vi "Destroy.vi"(8 "error in (no error)":errorcluster, 11 "Server in":refnum<class "Server.lvclass">) -> (0 "error out":errorcluster, 3 "Server out":refnum<class "Server.lvclass">)   [LabVIEW 2013, in "MQTT Server.lvlib" / "Server.lvclass"]
uses:
  Server.lvclass
  MQTT_Base/MQTT_Base.lvclass
  Server.lvclass/Server.ctl
  StoredSessions/StoredSessions.lvclass
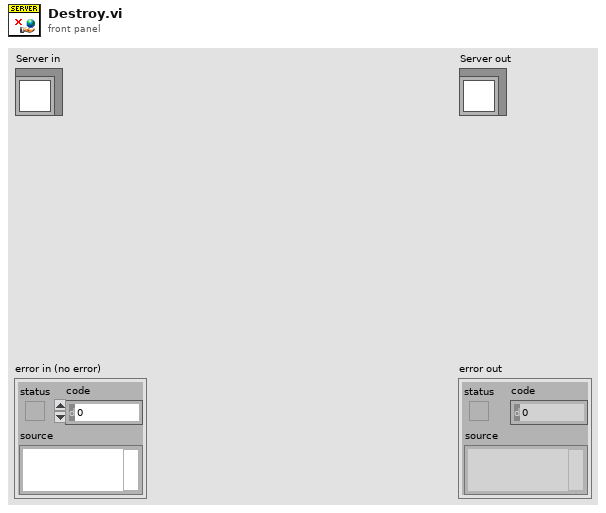
[diagram p1: front panel]
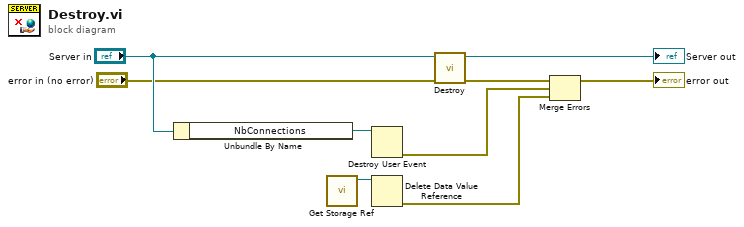
[diagram p0: block diagram]
diagram:
  n1 = Unbundle By Name("Server in") -> ("NbConnections"=w6:refnum<user-event>)
  n2 = call "Get Storage Ref.vi"() -> ("Storage"=w8:refnum<data-value>)  [unwired: 11 in]
  n3 = Destroy User Event(user event=w6) -> (error out=w1:errorcluster)  [unwired: 1 in]
  n4 = Delete Data Value Reference(data value reference=w8) -> (error out=w7:errorcluster)  [unwired: 1 in, 1 out]
  n5 = call-parent "Destroy.vi"("error in (no error)"="error in (no error)", "MQTT_Base in"="Server in") -> ("error out"=w3:errorcluster, "MQTT_Base out"=→"Server out":refnum<class "Server.lvclass">)  [unwired: 8 in]
  n6 = Merge Errors(w3, w1, w7) -> (→"error out":errorcluster)
